vi "Action - XNET CAN Reader with ID.vi"(7 "PackageID":i32, 8 "error in":errorcluster, 11 "CAN Configuration":T1={"CAN Interface"="CAN1", "XNET Cluster"="ManyXnetChannels", "#Signals"=0, "Sample Rate (Hz)"=100.0} {"Sample Rate (Hz)" format="%#_13g"}) -> (0 "error out":errorcluster)   [LabVIEW 2021, in "XNET-CAN-Signal-Logger.lvlib"]
uses:
  XNET-CAN-Signal-Logger.lvlib
  Typedef/Def-CAN Port Configuration.ctl
  Typedef/Def-Data Queue Type.ctl
  <vilib>/xnet/xnet.llb/XNET Create Session (Signal Input Waveform).vi
  <userlib>/_NEVSTOP/GlobalStop/_gStop.vi
  <vilib>/xnet/xnet.llb/XNET Read (Signal Waveform) .vi
  <resource>/objmgr/xnet.rc
  <userlib>/_NEVSTOP/GlobalStop/GSTOP.lvlib
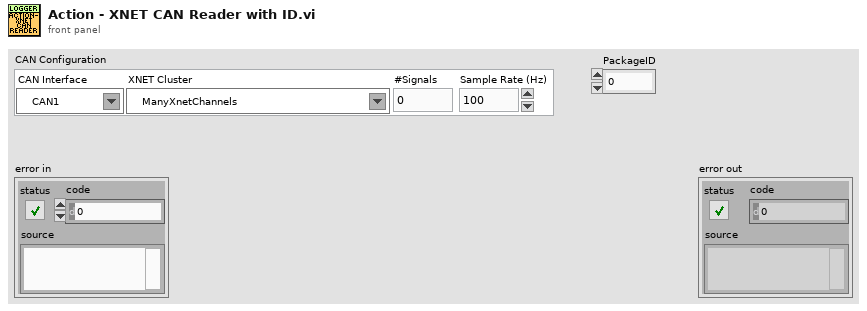
[diagram p1: front panel]
types:
  T1 = typedef "XNET-CAN-Signal-Logger.lvlib/Def-CAN Port Configuration.ctl" = cluster{"CAN Interface":refnum<k21>, "XNET Cluster":refnum<k21>, "#Signals":i32, "Sample Rate (Hz)":dbl}
  T2 = typedef "XNET-CAN-Signal-Logger.lvlib/Def-Data Queue Type.ctl" = cluster{"PackageID":i32, "Data":waveform(dbl)[]}
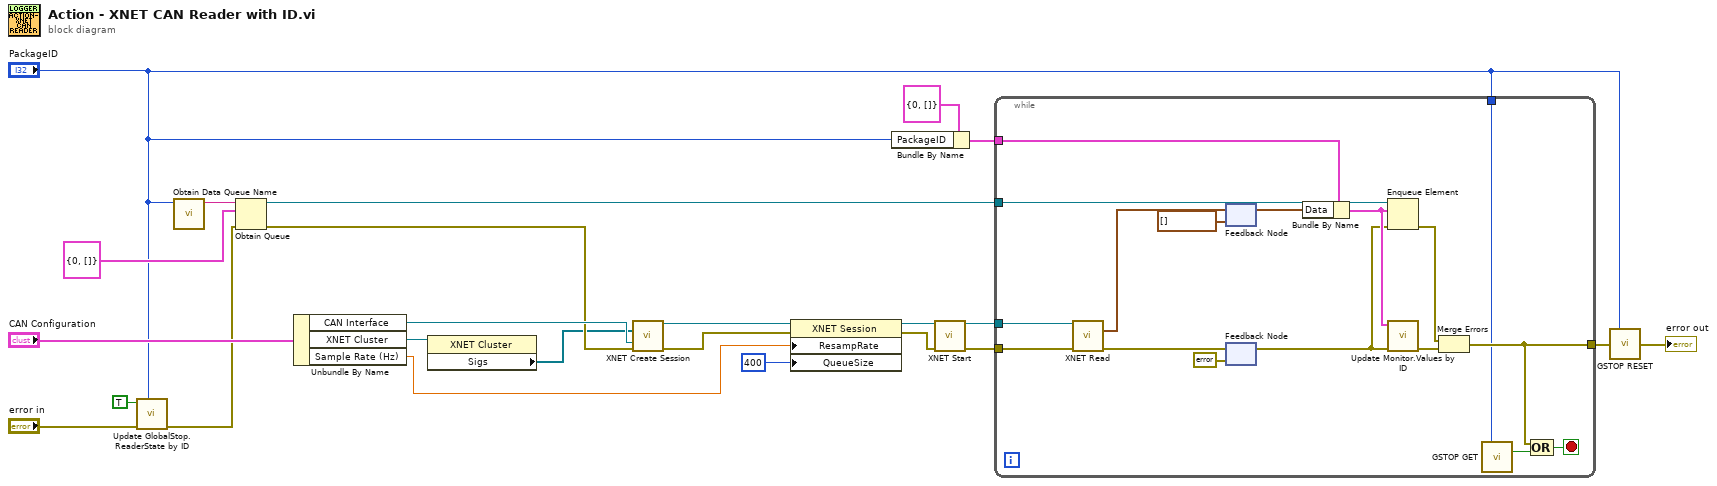
[diagram p0: block diagram]
diagram:
  n1 = call "Update GlobalStop.ReaderState by ID.vi"("PackageID"="PackageID", "error in"="error in", "RunState"=TRUE) -> ("error out"=w5:errorcluster)  [unwired: 8 in]
  n2 = call "Obtain Data Queue Name.vi"("PackageID"="PackageID") -> ("DataQueueName"=w4:string)  [unwired: 10 in]
  n3 = Obtain Queue(name (unnamed)=w4, element data type=T2 {"PackageID"=0, "Data"=[]} ("Data Queue Type"), error in (no error)=w5) -> (queue out=w12:refnum<queue>, error out=w11:errorcluster)  [unwired: 2 in, 1 out]
  n4 = Unbundle By Name("CAN Configuration") -> ("CAN Interface"=w18:refnum<k21>, "XNET Cluster"=w19:refnum<k21>, "Sample Rate (Hz)"=w9:dbl)
  n5 = property class="XNET Cluster"(reference=w19) -> ("Sigs"=w10:refnum<k21>[])  [unwired: 1 in, 2 out]
  n6 = call-poly <vilib>:"XNET Create Session.vi"("signal list"=w10, "interface"=w18, "error in (no error)"=w11) -> ("session out"=w24:refnum<k21>, "error out"=w23:errorcluster)  [unwired: 11 in]
  n7 = property class="XNET Session"(reference=w24, error in=w23, "ResampRate"=w9, "QueueSize"=u32 400 ("Queue Size")) -> (reference out=w22:refnum<k21>, error out=w21:errorcluster)
  n8 = Bundle By Name(cluster=T2 {"PackageID"=0, "Data"=[]} ("element"), "PackageID"="PackageID") -> (w14:T2)
  n9 = call <vilib>:"XNET Start.vi"("session in"=w22, "error in (no error)"=w21) -> ("session out"=w17:refnum<k21>, "error out"=w16:errorcluster)  [unwired: 12 in]
  n10 = while {
    tunnel: w12 -> [w40]
    tunnel: w17 -> [w41]
    tunnel: w16 -> [w37]
    tunnel: w14 -> [w39]
    tunnel: [w31] -> w3
    tunnel: "PackageID" -> [w25]
    stop <- w38 stop-if-true
    n11 = call-poly <vilib>:"XNET Read.vi"("session in"=w41, "error in (no error)"=w37) -> ("data"=w36:waveform(dbl)[], "error out"=w34:errorcluster)  [unwired: 11 in, 1 out]
    n12 = feedback-in #1(w36) -> ()
    n13 = feedback #1(waveform(dbl)[] [] ("data")) -> (w30:waveform(dbl)[])
    n14 = feedback-in #2(w34) -> ()
    n15 = feedback #2(errorcluster {"status"=FALSE, "code"=0, "source"=""} ("error out")) -> (w29:errorcluster)
    n16 = Bundle By Name(cluster=w39, "Data"=w30) -> (w35:T2)
    n17 = Enqueue Element(queue=w40, element=w35, error in (no error)=w29) -> (error out=w32:errorcluster)  [unwired: 1 in, 2 out]
    n18 = call "Update Monitor.Values by ID.vi"("error in"=w29, "Data"=w35) -> ("error out"=w33:errorcluster)  [unwired: 9 in]
    n19 = Merge Errors(w32, w33) -> (w31:errorcluster)
    n20 = call <userlib>:"GSTOP GET.vi"("index(-1 for All)"=w25) -> ("stop"=w26:bool)  [unwired: 13 in, 1 out]
    n21 = Compound Arithmetic op=OR(w31, w26) -> (w38:bool)
  }
  n22 = call <userlib>:"GSTOP RESET.vi"("index(-1 for All)"="PackageID", "error in (no error)"=w3) -> ("error out"=→"error out":errorcluster)  [unwired: 13 in]
